vi "rqcBob Configure Modulator.vi"(8 "error in":errorcluster, 9 "modulator.clock delay":fxp<+,4,4>, 10 "modulator.config":T1={"modulator.start"=1000, "modulator.stop"=2700}, 11 "FPGA reference in":refnum<k20>) -> (0 "error out":errorcluster, 3 "FPGA reference out":refnum<k20>)   [LabVIEW 2019]
uses:
  FPGA/rqcBob/Custom Controls/rqcBob Modulator Config.ctl
  <vilib>/Utility/error.llb/Error Cluster From Error Code.vi
  <vilib>/rvi/errors/niLvFpgaAdjustHostInterfaceError.vi
  <vilib>/rvi/interface/nirviReadWriteControl/nirviReadWriteControl.xnode
  NiFpgaLv.dll
  <vilib>/rvi/interface/Simulation/niFpgaSimulationCallBeginRW.vi
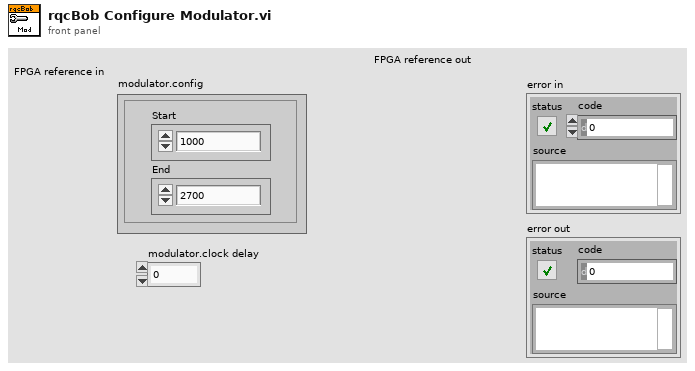
[diagram p1: front panel]
types:
  T1 = typedef "rqcBob Modulator Config.ctl" = cluster{"modulator.start":u16, "modulator.stop":u16}
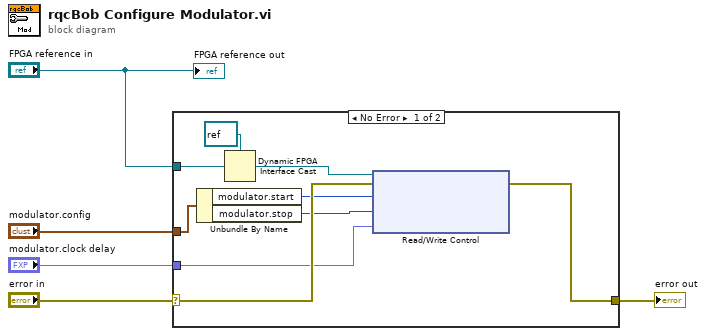
[diagram p0: block diagram]
diagram:
  n1 = case shown="No Error" "error in" {
    selector: "error in" -> [w14 w15]
    tunnel: [w13 w15] -> w3
    tunnel: "FPGA reference in" -> [w11 _]
    tunnel: "modulator.config" -> [w8 _]
    tunnel: "modulator.clock delay" -> [w9 _]
    frame No Error {
      n2 = Unbundle By Name(w8) -> ("modulator.start"=w7:u16, "modulator.stop"=w6:u16)
      n3 = Dynamic FPGA Interface Cast(Session In=refnum<k20> refnum ("FPGA Interface"), Type=w11) -> (Session Out=w10:refnum<k20>)
      n4 = xnode "Read/Write Control"("FPGA VI Reference In"=w10, "error in"=w14, "modulator.start"=w7, "modulator.stop"=w6, "modulator.clock delay"=w9) -> ("error out"=w13:errorcluster)  [unwired: 1 out]
    }
    frame Error {
    }
  }
  "error out" <- w3
  "FPGA reference out" <- "FPGA reference in"
